vi "实验1-2(子VI).vi"(9 "数值c":dbl, 10 "数值b":dbl, 11 "数值a":dbl) -> (3 "结果":dbl)   [LabVIEW 2018]
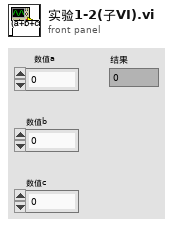
[diagram p1: front panel]
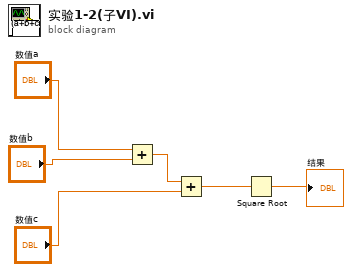
[diagram p0: block diagram]
diagram:
  n1 = Add(x="数值a", y="数值b") -> (x+y=w4:dbl)
  n2 = Add(x=w4, y="数值c") -> (x+y=w5:dbl)
  n3 = Square Root(x=w5) -> (sqrt(x)=→"结果":dbl)
